vi "comm wait for [string pattern].vi"(0 "Comm Handle":u32, 1 "timeout (10000)":u32=10000, 3 "Loop Delay (10)":u32=10, 5 "patterns":string[](array[string]), 9 "string in (\"\")":string, 11 "error in (no error)":errorcluster) -> (4 "dup Comm Handle":u32, 6 "match":bool, 8 "match substring":string, 10 "index found":i32, 12 "before match":string, 14 "after match":string, 15 "error out":errorcluster)   [LabVIEW 2017, in "lvserial.lvlib"]
doc: "This VI is receiving the data from the device and compares the data with the strings in 'pattern'. If one of the pattern matches, the VI returns 'match'=TRUE.\nAfter 'timeout' the 'match' is FALSE and all received data are lost.\n\nThe comparison is done by using the Match Pattern function of LabVIEW."
uses:
  lvserial.lvlib
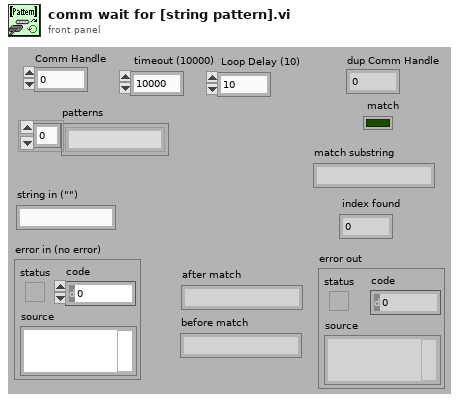
[diagram p1: front panel]
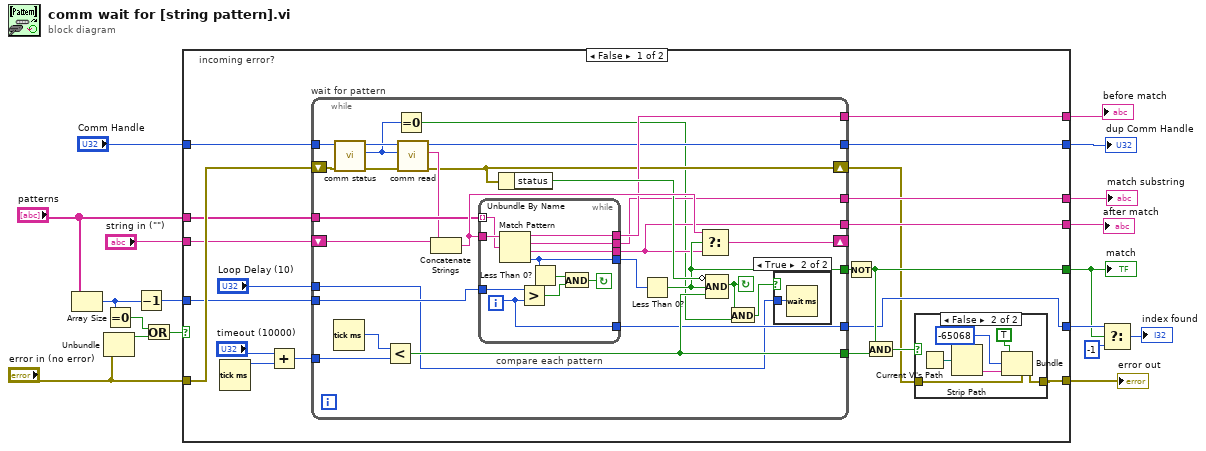
[diagram p0: block diagram]
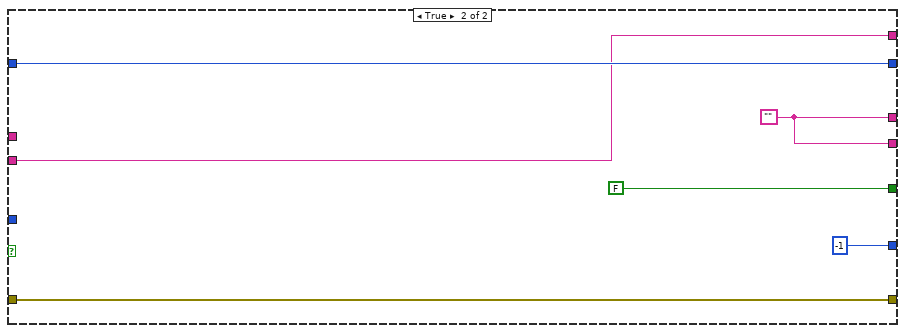
[diagram p4: hidden frame]
diagram:
  n1 = Array Size(array="patterns") -> (size(s)=w5:i32)
  n2 = Unbundle("error in (no error)") -> ("status"=w9:bool)  [unwired: 2 out]
  n3 = Equal To 0?(x=w5) -> (x = 0?=w7:bool)
  n4 = Decrement(x=w5) -> (x-1=w4:i32)
  n5 = Or(x=w7, y=w9) -> (x .or. y?=w8:bool)
  n6 = case "incoming error?" shown="False" w8 {
    tunnel: [w25 FALSE] -> w12
    tunnel: "error in (no error)" -> [w36 w90]
    tunnel: [w20 w90] -> w1
    tunnel: "Comm Handle" -> [w37 w88]
    tunnel: [w19 w88] -> w17
    tunnel: [w23 -1] -> w14
    tunnel: [w32 w86] -> w16
    tunnel: [w31 w85] -> w15
    tunnel: [w30 w86] -> w10
    tunnel: "patterns" -> [w29 _]
    tunnel: "string in (\"\")" -> [w28 w85]
    tunnel: w4 -> [w24 _]
    frame False {
      n7 = Tick Count (ms)() -> (millisecond timer value=w35:u32)
      n8 = Add(x="timeout (10000)", y=w35) -> (x+y=w38:u32)
      n9 = while "wait for pattern" {
        tunnel: [w50] -> w19
        tunnel: w24 -> [w51]
        tunnel: w29 -> [w52]
        tunnel: [w53] -> w30
        tunnel: [w54] -> w31
        tunnel: [w55] -> w32
        tunnel: [w56] -> w23
        tunnel: "Loop Delay (10)" -> [w44]
        tunnel: [w57] -> w27
        shift-left: w36 -> [w43]
        shift-right: [w48] -> w21
        tunnel: [w58] -> w26
        tunnel: w37 -> [w42]
        shift-left: w28 -> [w61]
        shift-right: [w62] -> _
        tunnel: w38 -> [w64]
        stop <- w47 continue-if-true
        n10 = Tick Count (ms)() -> (millisecond timer value=w65:u32)
        n11 = call "comm status.vi"("error in (no error)"=w43, "Comm Handle"=w42) -> ("error out"=w39:errorcluster, "In Queue"=w40:u32, "dup Comm Handle"=w41:u32)  [unwired: 7 out]
        n12 = Less?(x=w65, y=w64) -> (x < y?=w57:bool)
        n13 = Equal To 0?(x=w40) -> (x = 0?=w46:bool)
        n14 = call "comm read.vi"("error in (no error)"=w39, "requested byte count"=w40, "Comm Handle"=w41) -> ("error out"=w48:errorcluster, "string read"=w49:string, "dup Comm Handle"=w50:u32)  [unwired: 6 out]
        n15 = Concatenate Strings(w61, w49) -> (w60:string)
        n16 = while "compare each pattern" {
          tunnel: [w66] -> w53
          tunnel: [w67] -> w54
          tunnel: [w68] -> w56
          tunnel: w51 -> [w69]
          tunnel: w52 -> [w74] mode=indexing
          tunnel: [w73] -> w63
          tunnel: [w75] -> w55
          tunnel: w60 -> [w76]
          i -> [w68]
          stop <- w70 continue-if-true
          n17 = Match Pattern(string=w76, regular expression=w74) -> (before substring=w67:string, match substring=w66:string, after substring=w75:string, offset past match=w73:i32)  [unwired: 1 out]
          n18 = Greater?(x=w69, y=w68) -> (0:w71:bool)
          n19 = Less Than 0?(x=w73) -> (x < 0?=w72:bool)
          n20 = And(x=w72, y=w71) -> (x .and. y?=w70:bool)
        }
        n21 = Unbundle By Name(w48) -> ("status"=w59:bool)
        n22 = Less Than 0?(x=w63) -> (x < 0?=w58:bool)
        n23 = Select(t=w60, s=w58, f=w55) -> (s? t:f=w62:string)
        n24 = Compound Arithmetic op=AND(invert w59, w58, w57) -> (w47:bool)
        n25 = And(x=w47, y=w46) -> (x .and. y?=w45:bool)
        n26 = case shown="True" w45 {
          tunnel: w44 -> [_ w77]
          frame False {
          }
          frame True {
            n27 = Wait (ms)(milliseconds to wait=w77) -> ()  [unwired: 1 out]
          }
        }
      }
      n28 = Not(x=w26) -> (.not. x?=w25:bool)
      n29 = And(x=w25, y=w27) -> (x .and. y?=w22:bool)
      n30 = case shown="False" w22 {
        tunnel: w21 -> [w78 w84]
        tunnel: [w78 w83] -> w20
        frame True {
        }
        frame False {
          n31 = Current VI's Path() -> (path=w80:path)
          n32 = Strip Path(path=w80) -> (name=w81:string)  [unwired: 1 out]
          n33 = Bundle(cluster=w84, "status"=TRUE, "code"=-65068, "source"=w81) -> (w83:errorcluster)
        }
      }
    }
    frame True {
      w86 = ""
    }
  }
  "match" <- w12
  "dup Comm Handle" <- w17
  "after match" <- w16
  "before match" <- w15
  "match substring" <- w10
  "error out" <- w1
  n34 = Select(t=w14, s=w12, f=-1) -> (s? t:f=→"index found":i32)
